vi "Fläche.vi"(9 "Numeric 2":dbl, 10 "Numeric":dbl, 11 "error in (no error)":errorcluster) -> (1 "error out":errorcluster, 2 "Numeric 3":dbl)   [LabVIEW 2024]
doc: "Berechnet die Fläche von Rechtecken/Quadraten"
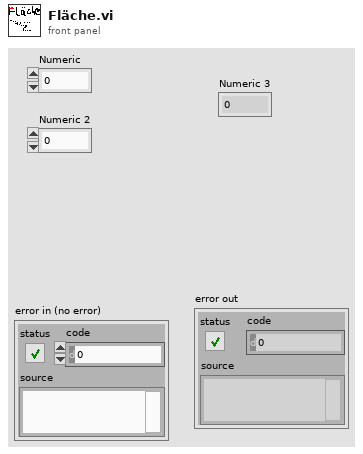
[diagram p1: front panel]
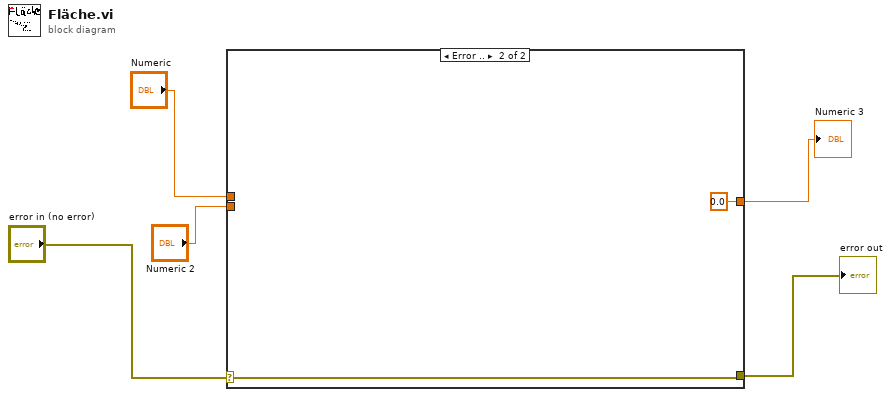
[diagram p0: block diagram]
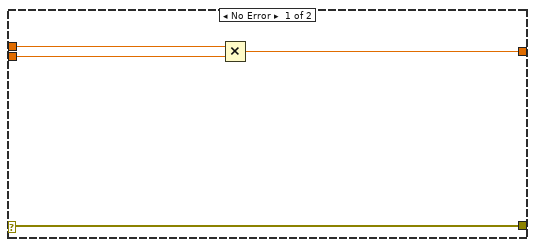
[diagram p2: hidden frame]
diagram:
  n1 = case shown="Error .." "error in (no error)" {
    selector: "error in (no error)" -> [w9 w11]
    tunnel: [w9 w11] -> w4
    tunnel: "Numeric" -> [w8 _]
    tunnel: "Numeric 2" -> [w7 _]
    tunnel: [w6 0.0] -> w1
    frame No Error {
      n2 = Multiply(x=w8, y=w7) -> (x*y=w6:dbl)
    }
    frame Error {
    }
  }
  "error out" <- w4
  "Numeric 3" <- w1
